vi "fgv_ctrl-ref.vi"(7 "cmd":T2, 8 "error in":errorcluster, 11 "output cluster":T1) -> (0 "error out":errorcluster, 3 "output cluster 2":T1)   [LabVIEW 2019]
uses:
  _ctrl/rw.ctl
  Durability/common/ref_all.ctl
  Durability/Capacitor/Judge_RC.ctl
  Durability/Breakdown-Spec.ctl
  _ctrl/DL950_config.ctl
  Durability/Capacitor/cap_config.ctl
panel:
  # "제어단 전압"
  # "출력단 전원"
  # "DL950"
  # "Discharge"
  # "Test Cycle"
  # "작동 설정"
  # "C 전압1"
  # "C 전압2"
  # "출력전압(+)"
  # "출력전압(-)"
  # "입력전류"
  # "출력전류"
  # "제어단"
  # "출력단"
  # "온도기준"
  # "제어단 전압"
  # "출력단 전원"
  # "DL950"
  # "Discharge"
  # "Test Cycle"
  # "작동 설정"
  # "C 전압1"
  # "C 전압2"
  # "출력전압(+)"
  # "출력전압(-)"
  # "입력전류"
  # "출력전류"
  # "제어단"
  # "출력단"
  # "온도기준"
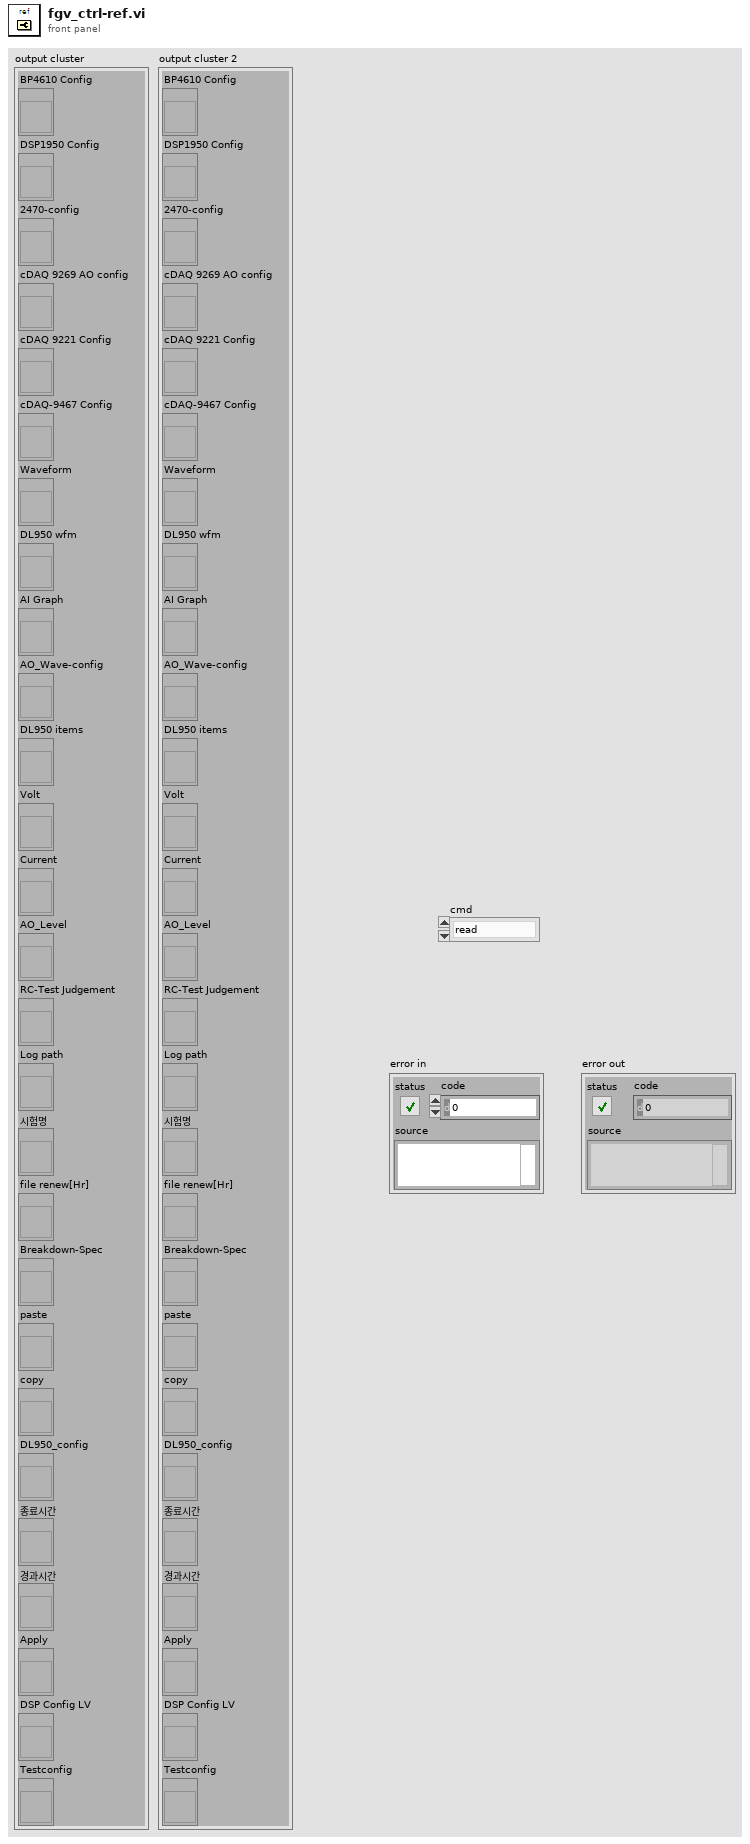
[diagram p1: front panel]
types:
  T1 = typedef "ref_all.ctl" = cluster{"BP4610 Config":refnum<vi>, "DSP1950 Config":refnum<vi>, "2470-config":refnum<vi>, "cDAQ 9269 AO config":refnum<vi>, "cDAQ 9221 Config":refnum<vi>, "cDAQ-9467 Config":refnum<vi>, "Waveform":refnum<vi>, "DL950 wfm":refnum<vi>, "AI Graph":refnum<vi>, "AO_Wave-config":refnum<vi>, "DL950 items":refnum<vi>, "Volt":refnum<vi>, "Current":refnum<vi>, "AO_Level":refnum<vi>, "RC-Test Judgement ":refnum<vi>, "Log path":refnum<vi>, "시험명":refnum<vi>, "file renew[Hr]":refnum<vi>, "Breakdown-Spec":refnum<vi>, "paste":refnum<vi>, "copy":refnum<vi>, "DL950_config":refnum<vi>, "종료시간":refnum<vi>, "경과시간":refnum<vi>, "Apply":refnum<vi>, "DSP Config LV ":refnum<vi>, "Testconfig":refnum<vi>}
  T2 = typedef "rw.ctl" = enum16{"read", "write"}
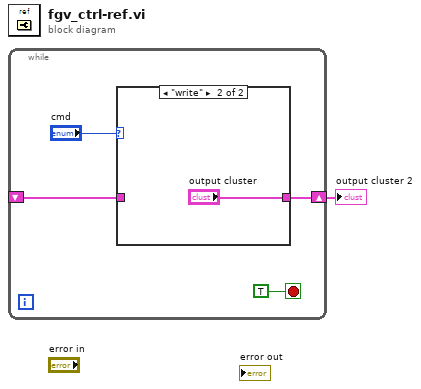
[diagram p0: block diagram]
diagram:
  n1 = while {
    shift-right: [w3] -> w1
    shift-left: _ -> [w2]
    stop <- TRUE stop-if-true
    n2 = case shown="\"write\"" "cmd" {
      tunnel: [w6 "output cluster"] -> w3
      tunnel: w2 -> [w6 _]
      frame "read", Default {
      }
      frame "write" {
      }
    }
  }
  "output cluster 2" <- w1
